vi "Sequence Editor.vi"() -> ()   [LabVIEW 2020, in "QuPMXdriver.lvlib"]
uses:
  QuPMXdriver.lvlib
  baab1036-9183-42e0-bbc8-3fcf3f36b3b7.vi
  QuP Multiplexer Control.vi
  <vilib>/Comparison/Equal/Equal Functor/Equal Functor.lvclass
panel:
  in  "clear sequence":bool
  in  "all timings to first one":bool
  in  "Sequence file path\n(file dialog if empty)":path=path "D:/martin/QPsw - github/QuPMX/seqtest"
  in  "Make test matrix":bool
  in  "delete last row":bool
  in  "hide":bool
  out "slaves connected":bool[](array[boolean])
  out "Sequence index":u32[](array[numeric]) min=1 max=255 step=1
  in  "Scrollbar":i32(c297)=1
  in  "Timing\ndelay":u32[](array[numeric]) min=1 max=255 step=1
  in  "Sequence":bool[][](array[boolean])
  in  "Load sq from file":bool
  in  "Save sq to file":bool
  # "Connected\nslaves"
  # "Slave index"
  # "1              2               3              4                5               6"
  # "Channel index"
  # "1     2       3      4       5      6      7       8      9     10     11    12"
  # "Sequence index"
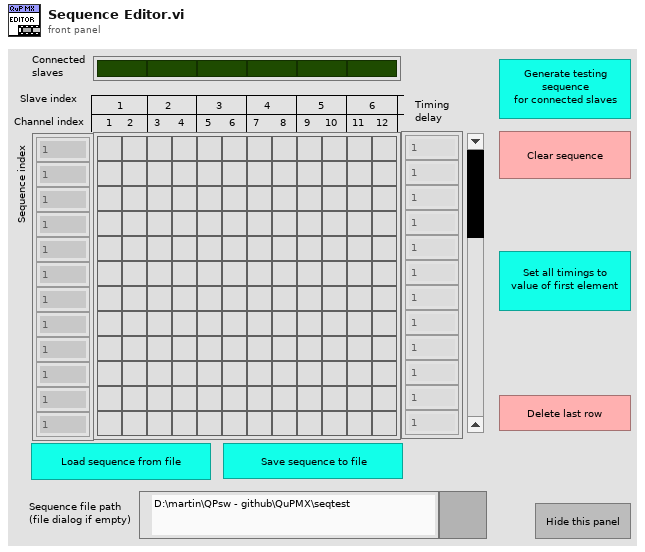
[diagram p1: front panel]
types:
  T1 = enum32{"Invalid", "Standard", "Closed", "Hidden", "Minimized", "Maximized"}
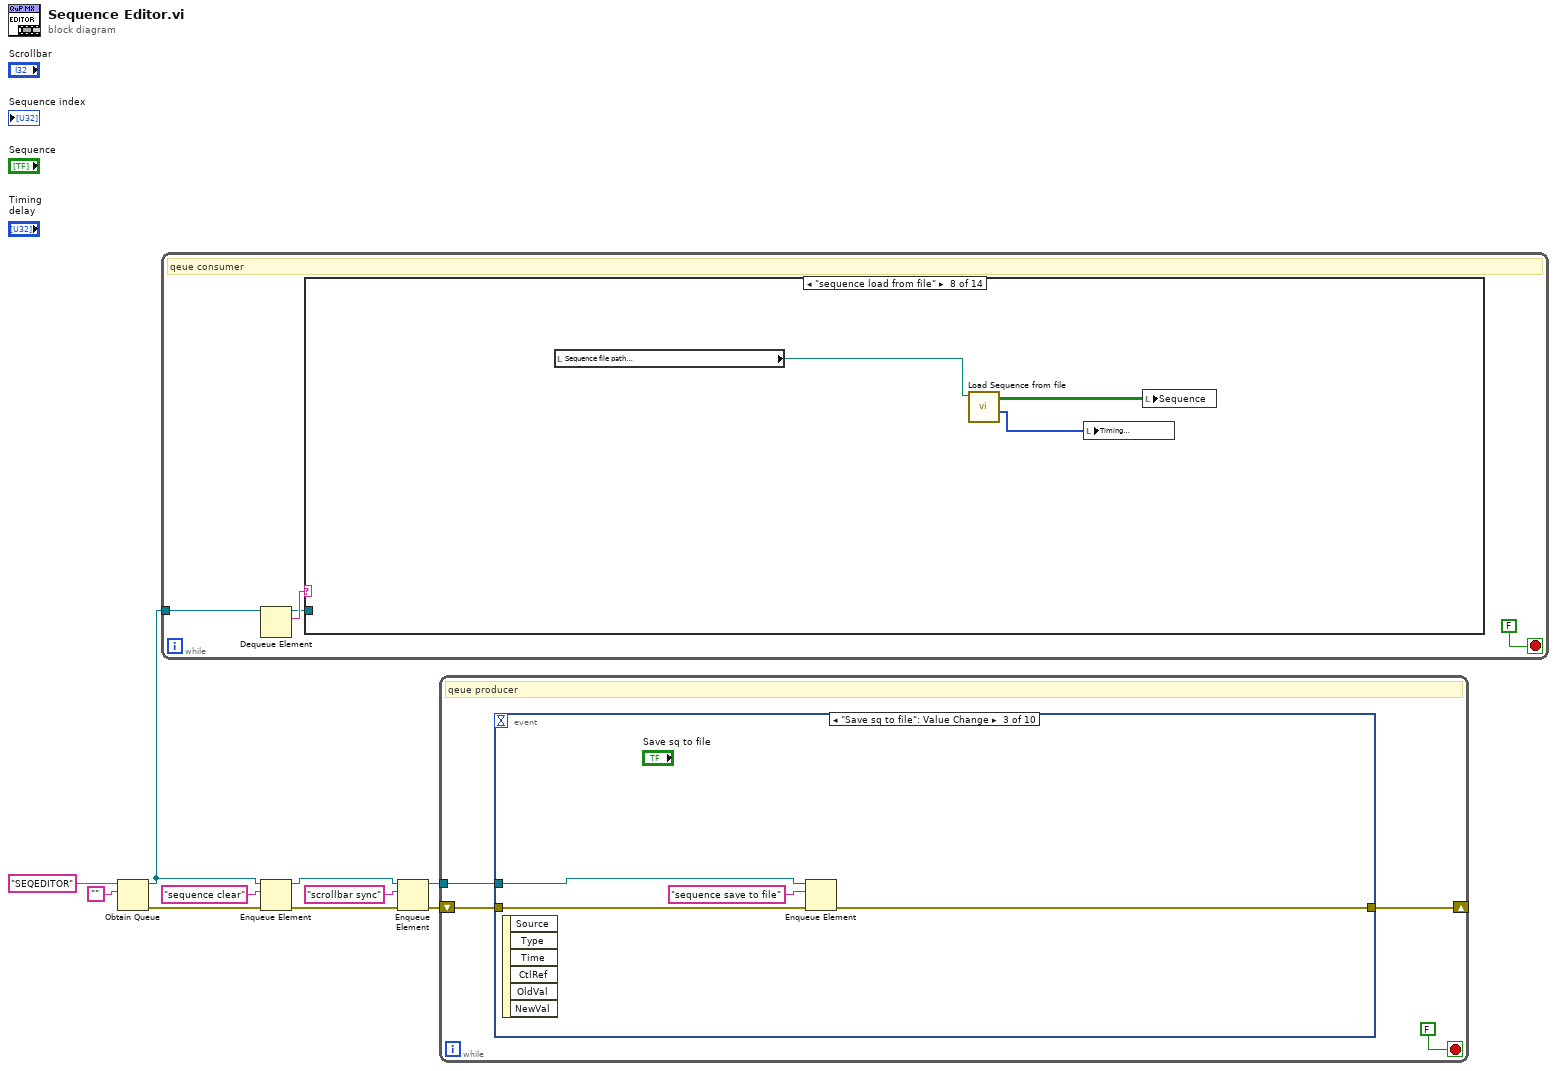
[diagram p0: block diagram]
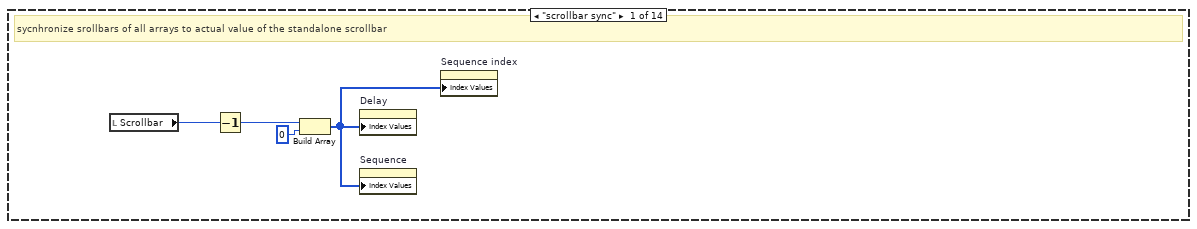
[diagram p2: hidden frame]
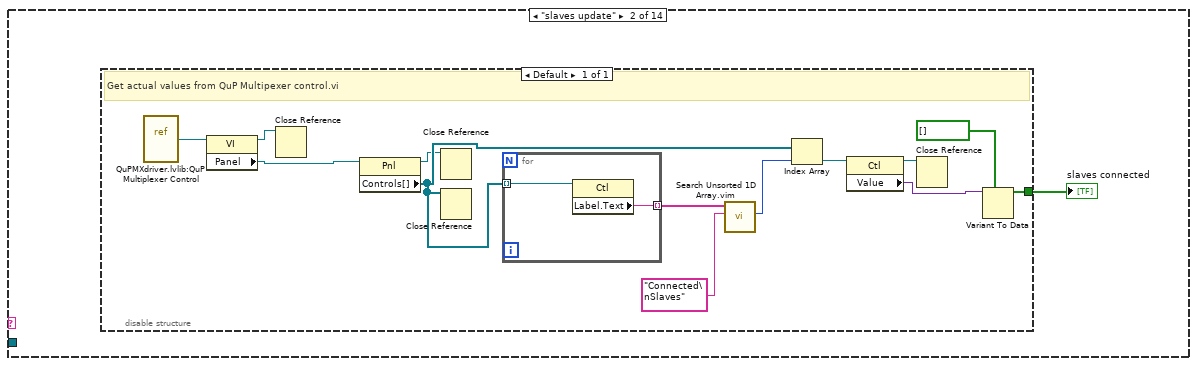
[diagram p3: hidden frame]
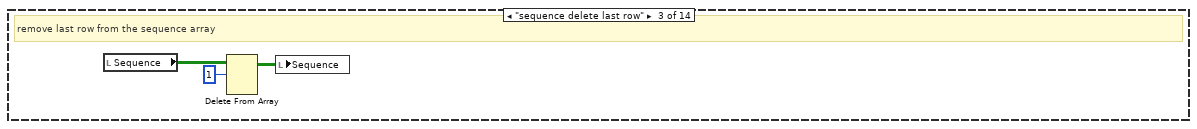
[diagram p4: hidden frame]
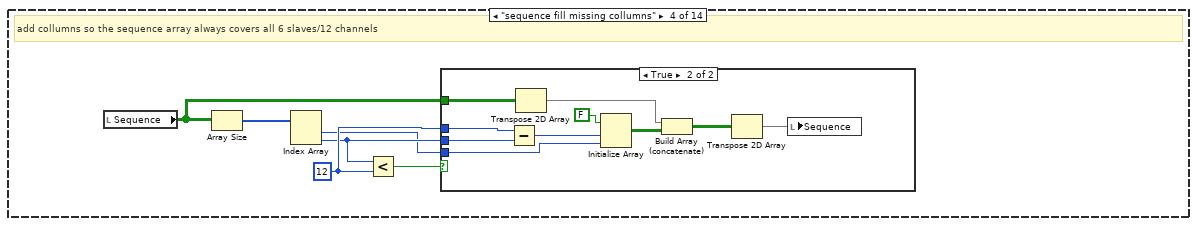
[diagram p5: hidden frame]
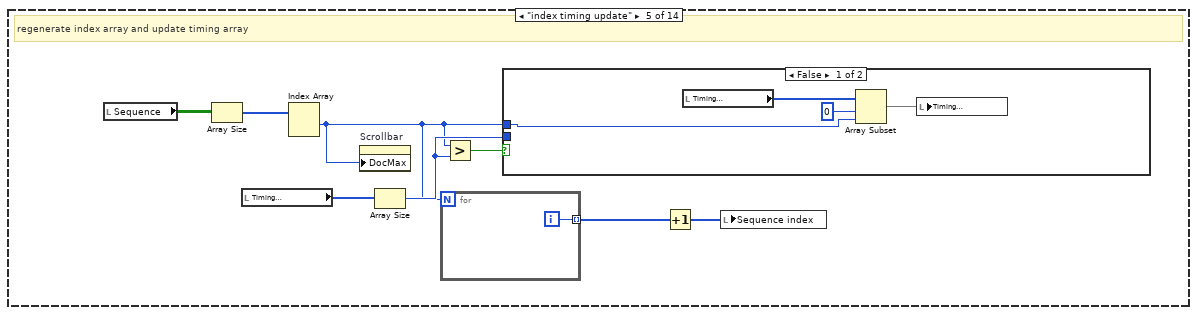
[diagram p7: hidden frame]
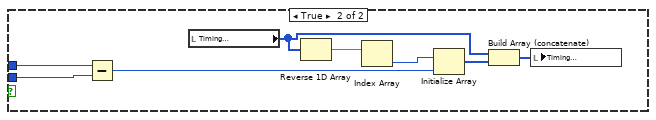
[diagram p8: hidden frame]
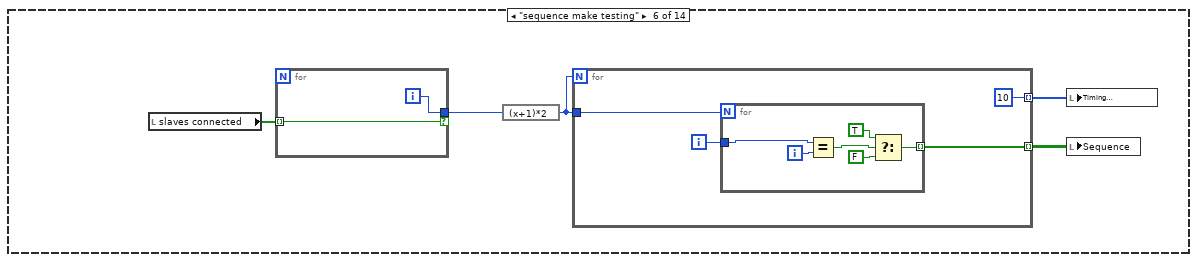
[diagram p9: hidden frame]
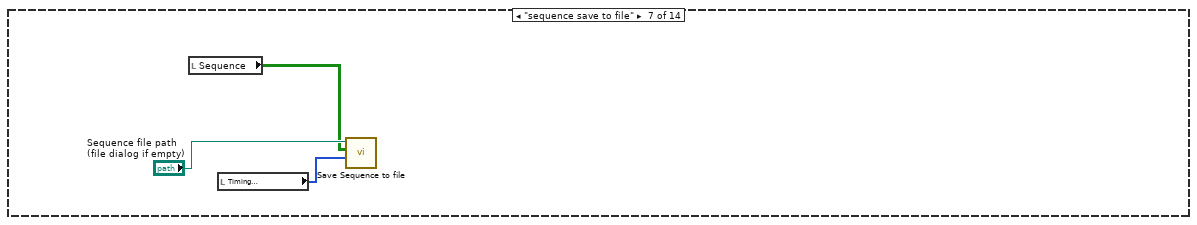
[diagram p10: hidden frame]
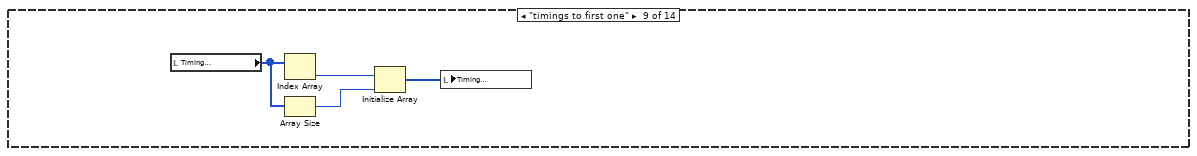
[diagram p11: hidden frame]
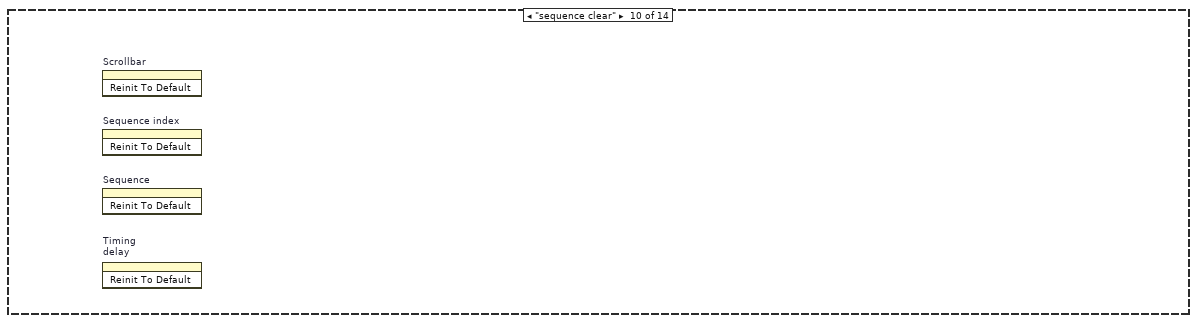
[diagram p12: hidden frame]
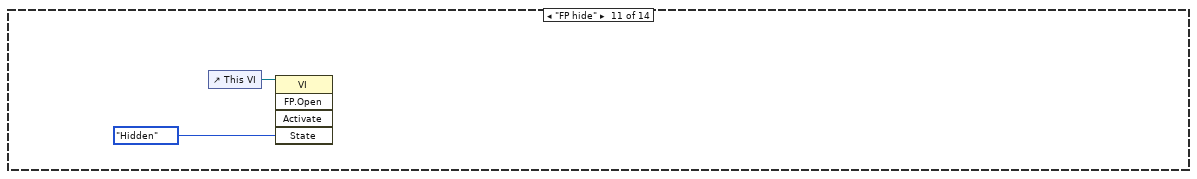
[diagram p13: hidden frame]
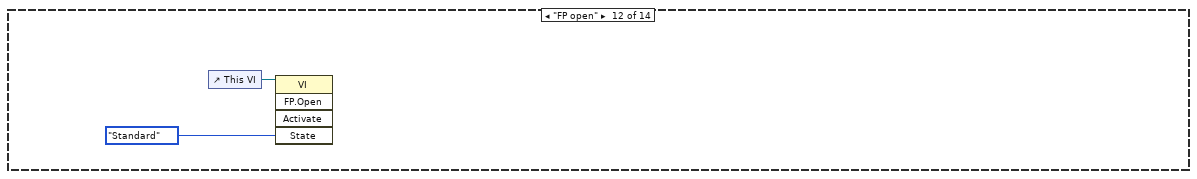
[diagram p14: hidden frame]
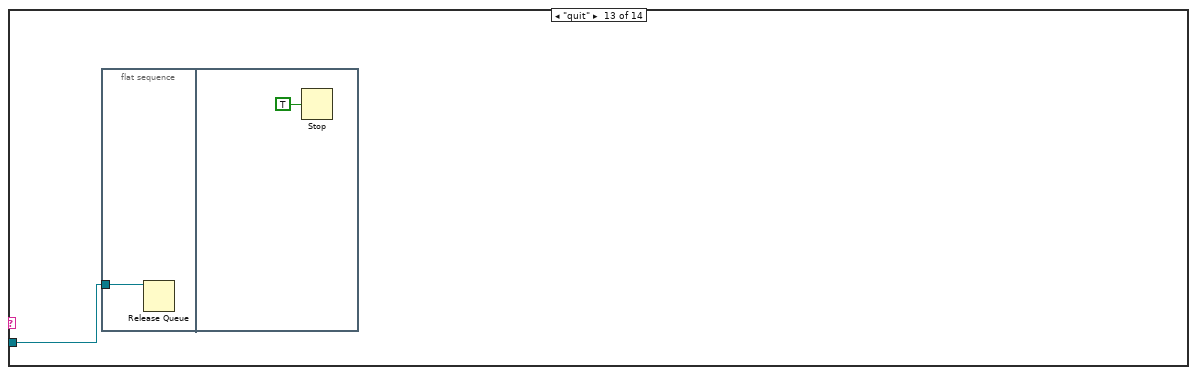
[diagram p15: hidden frame]
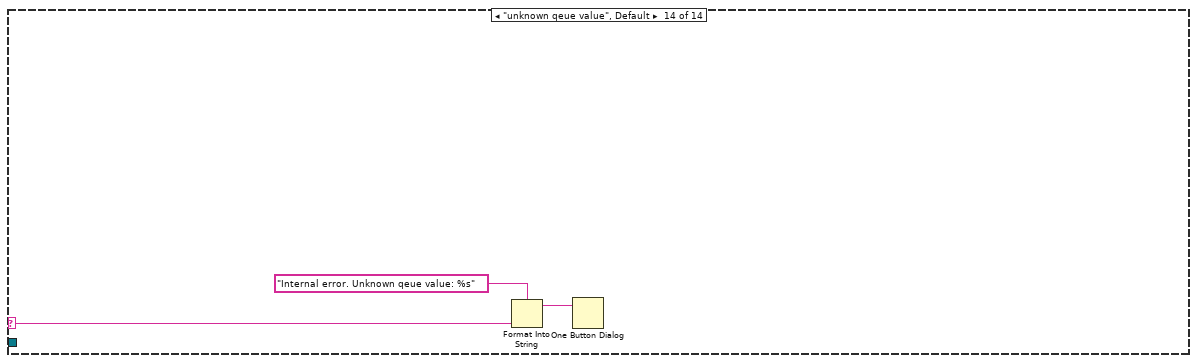
[diagram p16: hidden frame]
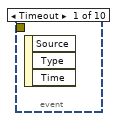
[diagram p17: hidden frame]
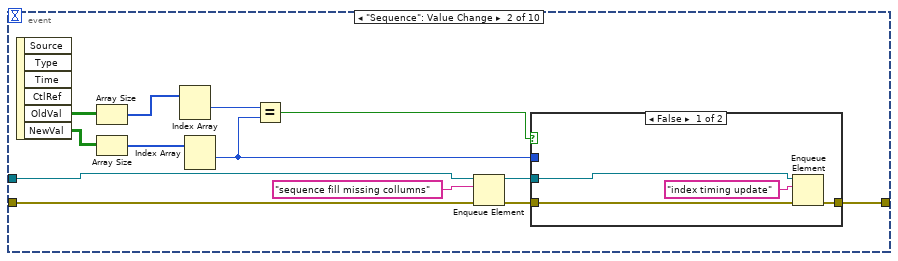
[diagram p18: hidden frame]
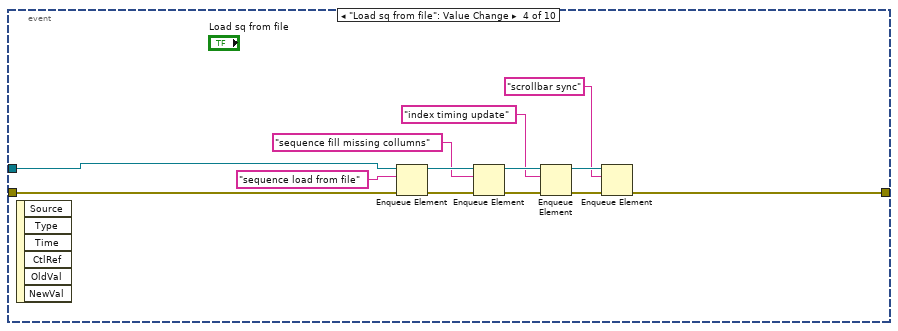
[diagram p20: hidden frame]
diagram:
  n1 = Obtain Queue(name (unnamed)="SEQEDITOR", element data type="" ("data (can be any type)")) -> (queue out=w9:refnum<queue>, error out=w8:errorcluster)  [unwired: 3 in, 1 out]
  n2 = while {
    tunnel: w9 -> [w14]
    stop <- FALSE stop-if-true
    # "qeue consumer"
    n3 = Dequeue Element(queue=w14) -> (queue out=w12:refnum<queue>, element=w13:string)  [unwired: 2 in, 2 out]
    n4 = case shown="\"sequence load from file\"" w13 {
      selector: w13 -> [_ _ _ _ _ _ _ _ _ _ _ _ _ w109]
      tunnel: w12 -> [_ _ _ _ _ _ _ _ _ _ _ _ w106 _]
      frame "scrollbar sync" {
        # "sycnhronize srollbars of all arrays to actual value of the standalone scrollbar"
        n5 = local read "Scrollbar"() -> (w15:i32)
        n6 = Decrement(x=w15) -> (x-1=w18:i32)
        n7 = Build Array(w18, u32 0) -> (w17:u32[])
        n8 = property on="Delay" class="Arr (strict)"("Index Values"=w17) -> ()  [unwired: 2 in, 2 out]
        n9 = property on="Sequence" class="Arr (strict)"("Index Values"=w17) -> ()  [unwired: 2 in, 2 out]
        n10 = property on="Sequence index" class="Arr (strict)"("Index Values"=w17) -> ()  [unwired: 2 in, 2 out]
      }
      frame "slaves update" {
        n11 = disable-structure shown="Default" {
          disable-tunnel: [w23] -> w19
          frame Enabled {
            # "Get actual values from QuP Multipexer control.vi"
            n12 = vi-ref "QuPMXdriver.lvlib:QuP Multiplexer Control.vi"() -> (w22:refnum<vi>)
            n13 = property class="VI"(reference=w22) -> (reference out=w21:refnum<vi>, "Panel"=w32:refnum<vi>)  [unwired: 1 in, 1 out]
            n14 = Close Reference(reference=w21) -> ()  [unwired: 1 in, 1 out]
            n15 = property class="Pnl"(reference=w32) -> (reference out=w24:refnum<vi>, "Controls[]"=w25:refnum<vi>[])  [unwired: 1 in, 1 out]
            n16 = Close Reference(reference=w24) -> ()  [unwired: 1 in, 1 out]
            n17 = Close Reference(reference=w25) -> ()  [unwired: 1 in, 1 out]
            n18 = for {
              tunnel: w25 -> [w34] mode=indexing
              tunnel: [w33] -> w27 mode=indexing
              n19 = property class="Ctl"(reference=w34) -> ("Label.Text"=w33:string)  [unwired: 1 in, 2 out]
            }
            n20 = call "Search Unsorted 1D Array.vim"("element"="Connected\nSlaves" ("Label.Text"), "unsorted 1D array"=w27) -> ("index of element"=w29:i32)  [unwired: 9 in]
            n21 = Index Array(array=w25, index=w29) -> (element=w30:refnum<vi>)
            n22 = property class="Ctl"(reference=w30) -> (reference out=w20:refnum<vi>, "Value"=w31:variant)  [unwired: 1 in, 1 out]
            n23 = Close Reference(reference=w20) -> ()  [unwired: 1 in, 1 out]
            n24 = Variant To Data(type=bool[] [], Variant=w31) -> (data=w23:bool[])  [unwired: 1 in, 1 out]
          }
        }
        "slaves connected" <- w19
      }
      frame "sequence delete last row" {
        # "remove last row from the sequence array"
        n25 = local read "Sequence"() -> (w36:bool[][])
        n26 = Delete From Array(array=w36, length=1) -> (array with subset deleted=w37:bool[][])  [unwired: 2 in, 1 out]
        n27 = local write "Sequence"(w37) -> ()
      }
      frame "sequence fill missing collumns" {
        w43 = 12 ("y")
        # "add collumns so the sequence array always covers all 6 slaves/12 channels"
        n28 = local read "Sequence"() -> (w40:bool[][])
        n29 = Array Size(array=w40) -> (size(s)=w41:i32[])
        n30 = Index Array(array=w41) -> (element #1=w38:i32, element #2=w39:i32)  [unwired: 2 in]
        n31 = Less?(x=w39, y=w43) -> (x < y?=w42:bool)
        n32 = case shown="True" w42 {
          tunnel: w40 -> [_ w48]
          tunnel: w38 -> [_ w52]
          tunnel: w39 -> [_ w51]
          tunnel: w43 -> [_ w50]
          frame False {
          }
          frame True {
            n33 = Subtract(x=w50, y=w51) -> (x-y=w49:i32)
            n34 = Transpose 2D Array(2D array=w48) -> (transposed array=w47:bool[][])
            n35 = Initialize Array(FALSE ("x < y?"), w49, w52) -> (w44:bool[][])
            n36 = Build Array (concatenate)(w47, w44) -> (w46:bool[][])
            n37 = Transpose 2D Array(2D array=w46) -> (transposed array=w45:bool[][])
            n38 = local write "Sequence"(w45) -> ()
          }
        }
      }
      frame "index timing update" {
        # "regenerate index array and update timing array"
        n39 = local read "Sequence"() -> (w55:bool[][])
        n40 = Array Size(array=w55) -> (size(s)=w56:i32[])
        n41 = local read "Timing\ndelay"() -> (w58:u32[])
        n42 = Index Array(array=w56) -> (element #1=w54:i32)  [unwired: 2 in, 1 out]
        n43 = property on="Scrollbar" class="Scroll (strict)"("DocMax"=w54) -> ()  [unwired: 2 in, 2 out]
        n44 = Array Size(array=w58) -> (size(s)=w59:i32)
        n45 = for {
          N: w54 -> [_]
          tunnel: [w74] -> w57 mode=indexing
          i -> [w74]
        }
        n46 = Greater?(x=w54, y=w59) -> (0:w60:bool)
        n47 = case shown="False" w60 {
          tunnel: w59 -> [_ w70]
          tunnel: w54 -> [w62 w69]
          frame False {
            n48 = local read "Timing\ndelay"() -> (w65:u32[])
            n49 = Array Subset(array=w65, index=0, length=w62) -> (w63:u32[])
            n50 = local write "Timing\ndelay"(w63) -> ()
          }
          frame True {
            n51 = Subtract(x=w69, y=w70) -> (x-y=w66:i32)
            n52 = local read "Timing\ndelay"() -> (w68:u32[])
            n53 = Reverse 1D Array(array=w68) -> (reversed array=w67:u32[])
            n54 = Index Array(array=w67) -> (element=w73:u32)  [unwired: 1 in]
            n55 = Initialize Array(w73, w66) -> (w72:u32[])
            n56 = Build Array (concatenate)(w68, w72) -> (w71:u32[])
            n57 = local write "Timing\ndelay"(w71) -> ()
          }
        }
        n58 = Increment(x=w57) -> (x+1=w61:i32[])
        n59 = local write "Sequence index"(w61) -> ()
      }
      frame "sequence make testing" {
        n60 = local read "slaves connected"() -> (w76:bool[])
        n61 = for {
          tunnel: w76 -> [w90] mode=indexing
          tunnel: [w91] -> w77 if=w90
          i -> [w91]
        }
        n62 = expression code="(x+1)*2"(w77) -> (w78:i32)
        n63 = for {
          N: w78 -> [_]
          tunnel: w78 -> [w83]
          tunnel: [w82] -> w79 mode=indexing
          tunnel: [10] -> w75 mode=indexing
          i -> [w81]
          n64 = for {
            N: w83 -> [_]
            tunnel: [w84] -> w82 mode=indexing
            tunnel: w81 -> [w89]
            i -> [w88]
            n65 = Equal?(x=w89, y=w88) -> (x = y?=w87:bool)
            n66 = Select(t=TRUE ("Boolean"), s=w87, f=FALSE ("Boolean")) -> (s? t:f=w84:bool)
          }
        }
        n67 = local write "Timing\ndelay"(w75) -> ()
        n68 = local write "Sequence"(w79) -> ()
      }
      frame "sequence save to file" {
        n69 = local read "Sequence"() -> (w93:bool[][])
        n70 = local read "Timing\ndelay"() -> (w92:u32[])
        n71 = call "Save Sequence to file.vi"("Timing\ndelay"=w92, "Sequence"=w93, "Sequence file path\n(file dialog if empty)"="Sequence file path\n(file dialog if empty)") -> ()  [unwired: 8 in, 1 out]
      }
      frame "sequence load from file" {
        n72 = local read "Sequence file path\n(file dialog if empty)"() -> (w95:path)
        n73 = call "Load Sequence from file.vi"("Sequence file path\n(file dialog if empty)"=w95) -> ("Timing\ndelay"=w97:u32[], "Sequence"=w96:bool[][])  [unwired: 8 in, 1 out]
        n74 = local write "Timing\ndelay"(w97) -> ()
        n75 = local write "Sequence"(w96) -> ()
      }
      frame "timings to first one" {
        n76 = local read "Timing\ndelay"() -> (w101:u32[])
        n77 = Index Array(array=w101) -> (element=w100:u32)  [unwired: 1 in]
        n78 = Array Size(array=w101) -> (size(s)=w99:i32)
        n79 = Initialize Array(w100, w99) -> (w98:u32[])
        n80 = local write "Timing\ndelay"(w98) -> ()
      }
      frame "sequence clear" {
        n81 = invoke on="Scrollbar" class="Scroll (strict)" method="Reinit To Default"() -> ()  [unwired: 3 in, 3 out]
        n82 = invoke on="Sequence index" class="Arr (strict)" method="Reinit To Default"() -> ()  [unwired: 3 in, 3 out]
        n83 = invoke on="Sequence" class="Arr (strict)" method="Reinit To Default"() -> ()  [unwired: 3 in, 3 out]
        n84 = invoke on="Timing\ndelay" class="Arr (strict)" method="Reinit To Default"() -> ()  [unwired: 3 in, 3 out]
      }
      frame "FP hide" {
        n85 = control-ref of="This VI"() -> (w102:refnum<vi>)
        n86 = invoke class="VI" method="FP.Open"(reference=w102, "State"=T1."Hidden") -> ()  [unwired: 3 in, 5 out]
      }
      frame "FP open" {
        n87 = control-ref of="This VI"() -> (w104:refnum<vi>)
        n88 = invoke class="VI" method="FP.Open"(reference=w104, "State"=T1."Standard") -> ()  [unwired: 3 in, 5 out]
      }
      frame "quit" {
        n89 = flat-sequence {
          tunnel: w106 -> [w107]
          frame #0 {
            n90 = Release Queue(queue=w107) -> ()  [unwired: 2 in, 3 out]
          }
          frame #1 {
            n91 = Stop(stop? (T)=TRUE) -> ()
          }
        }
      }
      frame "unknown qeue value", Default {
        n92 = Format Into String(format string="Internal error. Unknown qeue value: %s", w109) -> (resulting string=w111:string)  [unwired: 2 in, 1 out]
        n93 = One Button Dialog(message=w111) -> ()  [unwired: 1 in, 1 out]
      }
    }
  }
  n94 = Enqueue Element(queue=w9, element="sequence clear", error in (no error)=w8) -> (queue out=w5:refnum<queue>, error out=w4:errorcluster)  [unwired: 1 in, 1 out]
  n95 = Enqueue Element(queue=w5, element="scrollbar sync", error in (no error)=w4) -> (queue out=w2:refnum<queue>, error out=w3:errorcluster)  [unwired: 1 in, 1 out]
  n96 = while {
    shift-right: [w115] -> _
    shift-left: w3 -> [w114]
    tunnel: w2 -> [w113]
    stop <- FALSE stop-if-true
    # "qeue producer"
    n97 = event shown="[2] \"Save sq to file\": Value Change" {
      selector: _ -> [_ _ _ _ _ _ _ _ _ _]
      dyn-events: _ -> [_ _ _ _ _ _ _ _ _ _]
      timeout: _ -> [_ _ _ _ _ _ _ _ _ _]
      tunnel: [_ w116 w135 w138 w152 w158 w168 w175 w181 w186] -> w115
      tunnel: w114 -> [_ w120 w137 w148 w156 w159 w174 w176 w184 w187]
      tunnel: w113 -> [_ w121 w136 w149 w155 w160 w167 w178 w183 w188]
      event Timeout {
        n98 = event-data() -> ()  [unwired: 1 in, 3 out]
      }
      event "Sequence": Value Change {
        n99 = event-data() -> ("OldVal"=w126:bool[][], "NewVal"=w123:bool[][])  [unwired: 1 in, 4 out]
        n100 = Array Size(array=w126) -> (size(s)=w127:i32[])
        n101 = Array Size(array=w123) -> (size(s)=w128:i32[])
        n102 = Index Array(array=w127) -> (element #1=w125:i32)  [unwired: 2 in, 1 out]
        n103 = Index Array(array=w128) -> (element #1=w122:i32)  [unwired: 2 in, 1 out]
        n104 = Equal?(x=w125, y=w122) -> (x = y?=w124:bool)
        n105 = Enqueue Element(queue=w121, element="sequence fill missing collumns", error in (no error)=w120) -> (queue out=w118:refnum<queue>, error out=w117:errorcluster)  [unwired: 1 in, 1 out]
        n106 = case shown="False" w124 {
          tunnel: w122 -> [_ _]
          tunnel: w118 -> [w131 _]
          tunnel: w117 -> [w130 w133]
          tunnel: [w129 w133] -> w116
          frame False {
            n107 = Enqueue Element(queue=w131, element="index timing update", error in (no error)=w130) -> (error out=w129:errorcluster)  [unwired: 1 in, 2 out]
          }
          frame True {
          }
        }
      }
      event "Save sq to file": Value Change {
        n108 = event-data() -> ()  [unwired: 1 in, 6 out]
        n109 = Enqueue Element(queue=w136, element="sequence save to file", error in (no error)=w137) -> (error out=w135:errorcluster)  [unwired: 1 in, 2 out]
      }
      event "Load sq from file": Value Change {
        n110 = event-data() -> ()  [unwired: 1 in, 6 out]
        n111 = Enqueue Element(queue=w149, element="sequence load from file", error in (no error)=w148) -> (queue out=w147:refnum<queue>, error out=w139:errorcluster)  [unwired: 1 in, 1 out]
        n112 = Enqueue Element(queue=w147, element="sequence fill missing collumns", error in (no error)=w139) -> (queue out=w146:refnum<queue>, error out=w140:errorcluster)  [unwired: 1 in, 1 out]
        n113 = Enqueue Element(queue=w146, element="index timing update", error in (no error)=w140) -> (queue out=w145:refnum<queue>, error out=w141:errorcluster)  [unwired: 1 in, 1 out]
        n114 = Enqueue Element(queue=w145, element="scrollbar sync", error in (no error)=w141) -> (error out=w138:errorcluster)  [unwired: 1 in, 2 out]
      }
      event "delete last row": Value Change {
        n115 = event-data() -> ()  [unwired: 1 in, 6 out]
        n116 = Enqueue Element(queue=w155, element="sequence delete last row", error in (no error)=w156) -> (queue out=w154:refnum<queue>, error out=w153:errorcluster)  [unwired: 1 in, 1 out]
        n117 = Enqueue Element(queue=w154, element="index timing update", error in (no error)=w153) -> (error out=w152:errorcluster)  [unwired: 1 in, 2 out]
      }
      event "Scrollbar": Value Change {
        n118 = event-data() -> ()  [unwired: 1 in, 6 out]
        n119 = Enqueue Element(queue=w160, element="scrollbar sync", error in (no error)=w159) -> (error out=w158:errorcluster)  [unwired: 1 in, 2 out]
      }
      event "Make test matrix": Value Change {
        n120 = event-data() -> ()  [unwired: 1 in, 6 out]
        n121 = Enqueue Element(queue=w167, element="sequence make testing", error in (no error)=w174) -> (queue out=w164:refnum<queue>, error out=w166:errorcluster)  [unwired: 1 in, 1 out]
        n122 = Enqueue Element(queue=w164, element="sequence fill missing collumns", error in (no error)=w166) -> (queue out=w163:refnum<queue>, error out=w165:errorcluster)  [unwired: 1 in, 1 out]
        n123 = Enqueue Element(queue=w163, element="index timing update", error in (no error)=w165) -> (queue out=w170:refnum<queue>, error out=w169:errorcluster)  [unwired: 1 in, 1 out]
        n124 = Enqueue Element(queue=w170, element="scrollbar sync", error in (no error)=w169) -> (error out=w168:errorcluster)  [unwired: 1 in, 2 out]
      }
      event "all timings to first one": Value Change {
        n125 = event-data() -> ()  [unwired: 1 in, 6 out]
        n126 = Enqueue Element(queue=w178, element="timings to first one", error in (no error)=w176) -> (error out=w175:errorcluster)  [unwired: 1 in, 2 out]
      }
      event "clear sequence": Value Change {
        n127 = event-data() -> ()  [unwired: 1 in, 6 out]
        n128 = Enqueue Element(queue=w183, element="sequence clear", error in (no error)=w184) -> (queue out=w180:refnum<queue>, error out=w182:errorcluster)  [unwired: 1 in, 1 out]
        n129 = Enqueue Element(queue=w180, element="scrollbar sync", error in (no error)=w182) -> (error out=w181:errorcluster)  [unwired: 1 in, 2 out]
      }
      event "hide": Value Change {
        n130 = event-data() -> ()  [unwired: 1 in, 6 out]
        n131 = Enqueue Element(queue=w188, element="FP hide", error in (no error)=w187) -> (error out=w186:errorcluster)  [unwired: 1 in, 2 out]
      }
    }
  }
